vi "数据读取判断.vi"() -> (0 "error out":errorcluster, 1 "connection ID":refnum<k5>, 2 "判断错误":bool)   [LabVIEW 2018]
panel:
  out "服务器IP":string
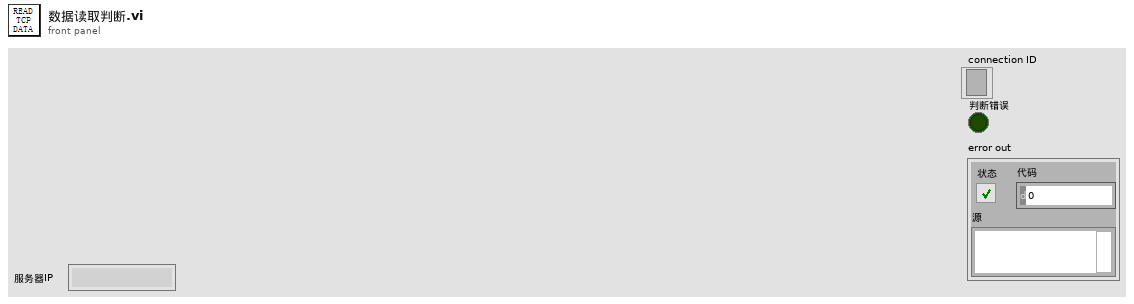
[diagram p1: front panel]
types:
  T1 = enum16{"Standard", "Buffered", "CRLF", "Immediate"}
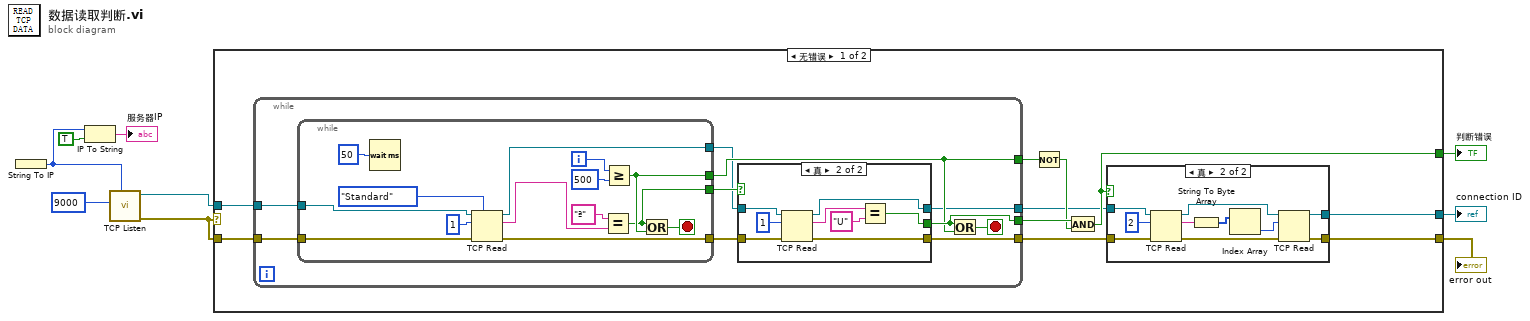
[diagram p0: block diagram]
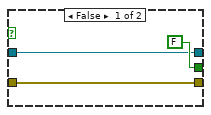
[diagram p3: hidden frame]
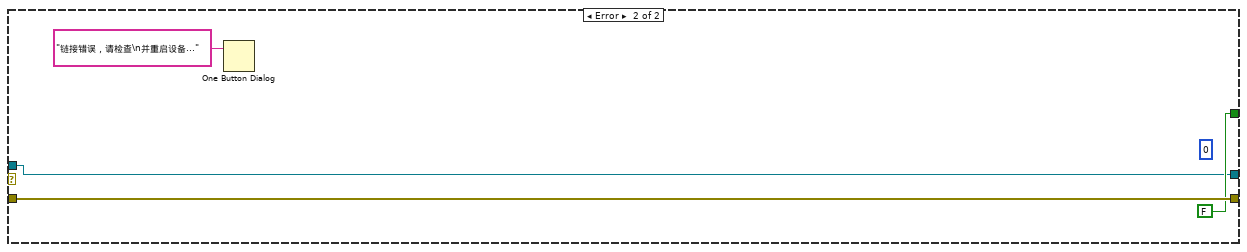
[diagram p4: hidden frame]
diagram:
  n1 = String To IP() -> (0:w6:u32)  [unwired: 1 in]
  n2 = IP To String(1:TRUE ("句点符号？(F)"), 2:w6) -> (0:→"服务器IP":string)
  n3 = call <vilib>:"TCP Listen.vi"("net address"=w6, "port"=u16 9000) -> ("error out"=w5:errorcluster, "connection ID"=w4:refnum<k5>)  [unwired: 5 in, 3 out]
  n4 = case shown="无错误" w5 {
    tunnel: w5 -> [w19 w70]
    tunnel: [w17 w70] -> w1
    tunnel: [w13 FALSE] -> w2
    tunnel: w4 -> [w12 w67]
    tunnel: [w10 w67] -> w3
    frame No Error {
      n5 = while {
        tunnel: w19 -> [w41]
        tunnel: [w39] -> w18
        tunnel: [w38] -> w16
        tunnel: [w36] -> w14
        tunnel: w12 -> [w34]
        tunnel: [w32] -> w11
        stop <- w37 stop-if-true
        n6 = while {
          tunnel: w41 -> [w58]
          tunnel: [w55] -> w40
          tunnel: [w63] -> w36
          tunnel: [w56] -> w35
          tunnel: w34 -> [w59]
          tunnel: [w54] -> w33
          i -> [w62]
          stop <- w65 stop-if-true
          n7 = Wait (ms)(milliseconds to wait=u32 50 ("等待时间（毫秒）")) -> ()  [unwired: 1 out]
          n8 = TCP Read(connection ID=w59, bytes to read=1 ("读取的字节"), error in (no error)=w58, 7:T1."Standard" ("模式（标准）")) -> (connection ID out=w54:refnum<k5>, data out=w53:string, error out=w55:errorcluster)  [unwired: 1 in]
          n9 = Equal?(x="ª", y=w53) -> (x = y?=w56:bool)
          n10 = Greater Or Equal?(x=w62, y=500) -> (x >= y?=w63:bool)
          n11 = Or(x=w56, y=w63) -> (x .or. y?=w65:bool)
        }
        n12 = case shown="真" w35 {
          tunnel: w40 -> [w44 w50]
          tunnel: [w44 w46] -> w39
          tunnel: [FALSE w51] -> w38
          tunnel: w33 -> [w42 w48]
          tunnel: [w42 w45] -> w32
          frame False {
          }
          frame True {
            n13 = TCP Read(connection ID=w48, bytes to read=u32 1 ("字节总数"), error in (no error)=w50) -> (connection ID out=w45:refnum<k5>, data out=w47:string, error out=w46:errorcluster)  [unwired: 2 in]
            n14 = Equal?(x=w47, y="U") -> (x = y?=w51:bool)
          }
        }
        n15 = Or(x=w38, y=w36) -> (x .or. y?=w37:bool)
      }
      n16 = Not(x=w14) -> (.not. x?=w15:bool)
      n17 = And(x=w16, y=w15) -> (x .and. y?=w13:bool)
      n18 = case shown="真" w13 {
        tunnel: w18 -> [w21 w30]
        tunnel: [w21 w28] -> w17
        tunnel: w11 -> [w20 w26]
        tunnel: [w20 w25] -> w10
        frame False {
        }
        frame True {
          n19 = TCP Read(connection ID=w26, bytes to read=u32 2 ("字节总数"), error in (no error)=w30) -> (connection ID out=w27:refnum<k5>, data out=w22:string, error out=w29:errorcluster)  [unwired: 2 in]
          n20 = String To Byte Array(string=w22) -> (unsigned byte array=w31:u8[])
          n21 = Index Array(array=w31) -> (element=w23:u8)  [unwired: 1 in]
          n22 = TCP Read(connection ID=w27, bytes to read=w23, error in (no error)=w29) -> (connection ID out=w25:refnum<k5>, error out=w28:errorcluster)  [unwired: 2 in, 1 out]
        }
      }
    }
    frame Error {
      (unwired) u8 0
      n23 = One Button Dialog(message="链接错误，请检查\n并重启设备..." ("消息")) -> ()  [unwired: 1 in, 1 out]
    }
  }
  "connection ID" <- w3
  "判断错误" <- w2
  "error out" <- w1
